vi "code rev.vi"(11 "Dashboard Revision":string) -> (0 "Found Revision":bool, 3 "Code Revision":string)   [LabVIEW 2015]
uses:
  <vilib>/Rock Robotics/Network Tables/NT Read String.vi
  <vilib>/Rock Robotics/Network Tables/NT Write String.vi
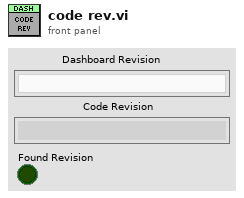
[diagram p1: front panel]
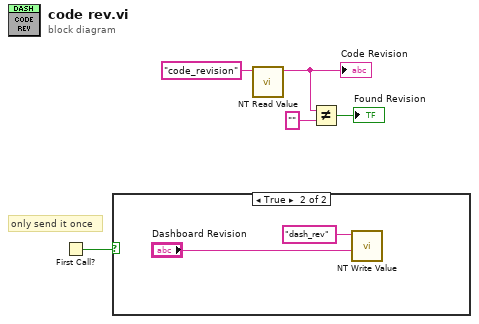
[diagram p0: block diagram]
diagram:
  # "only send it once"
  n1 = First Call?() -> (First Call?: T/F=w1:bool)
  n2 = case shown="True" w1 {
    frame False {
    }
    frame True {
      n3 = call-poly <vilib>:"NT Write Value.vi"("String"="Dashboard Revision", "Name"="dash_rev") -> ()  [unwired: 9 in, 1 out]
    }
  }
  n4 = call-poly <vilib>:"NT Read Value.vi"("Name"="code_revision") -> ("String"=w4:string)  [unwired: 9 in, 1 out]
  "Code Revision" <- w4
  n5 = Not Equal?(x=w4, y="") -> (x != y?=→"Found Revision":bool)
